vi "subVI_Mono2Go2Pos.vi"(2 "ESP300 Error":errorcluster, 3 "Postion (Unit)":dbl, 4 "ESP 300 COM Port":refnum<visa-resource-name>="COM4" caption="COM Port") -> (0 "error out":errorcluster, 1 "VISA resource name out":refnum<visa-resource-name>)   [LabVIEW 2019]
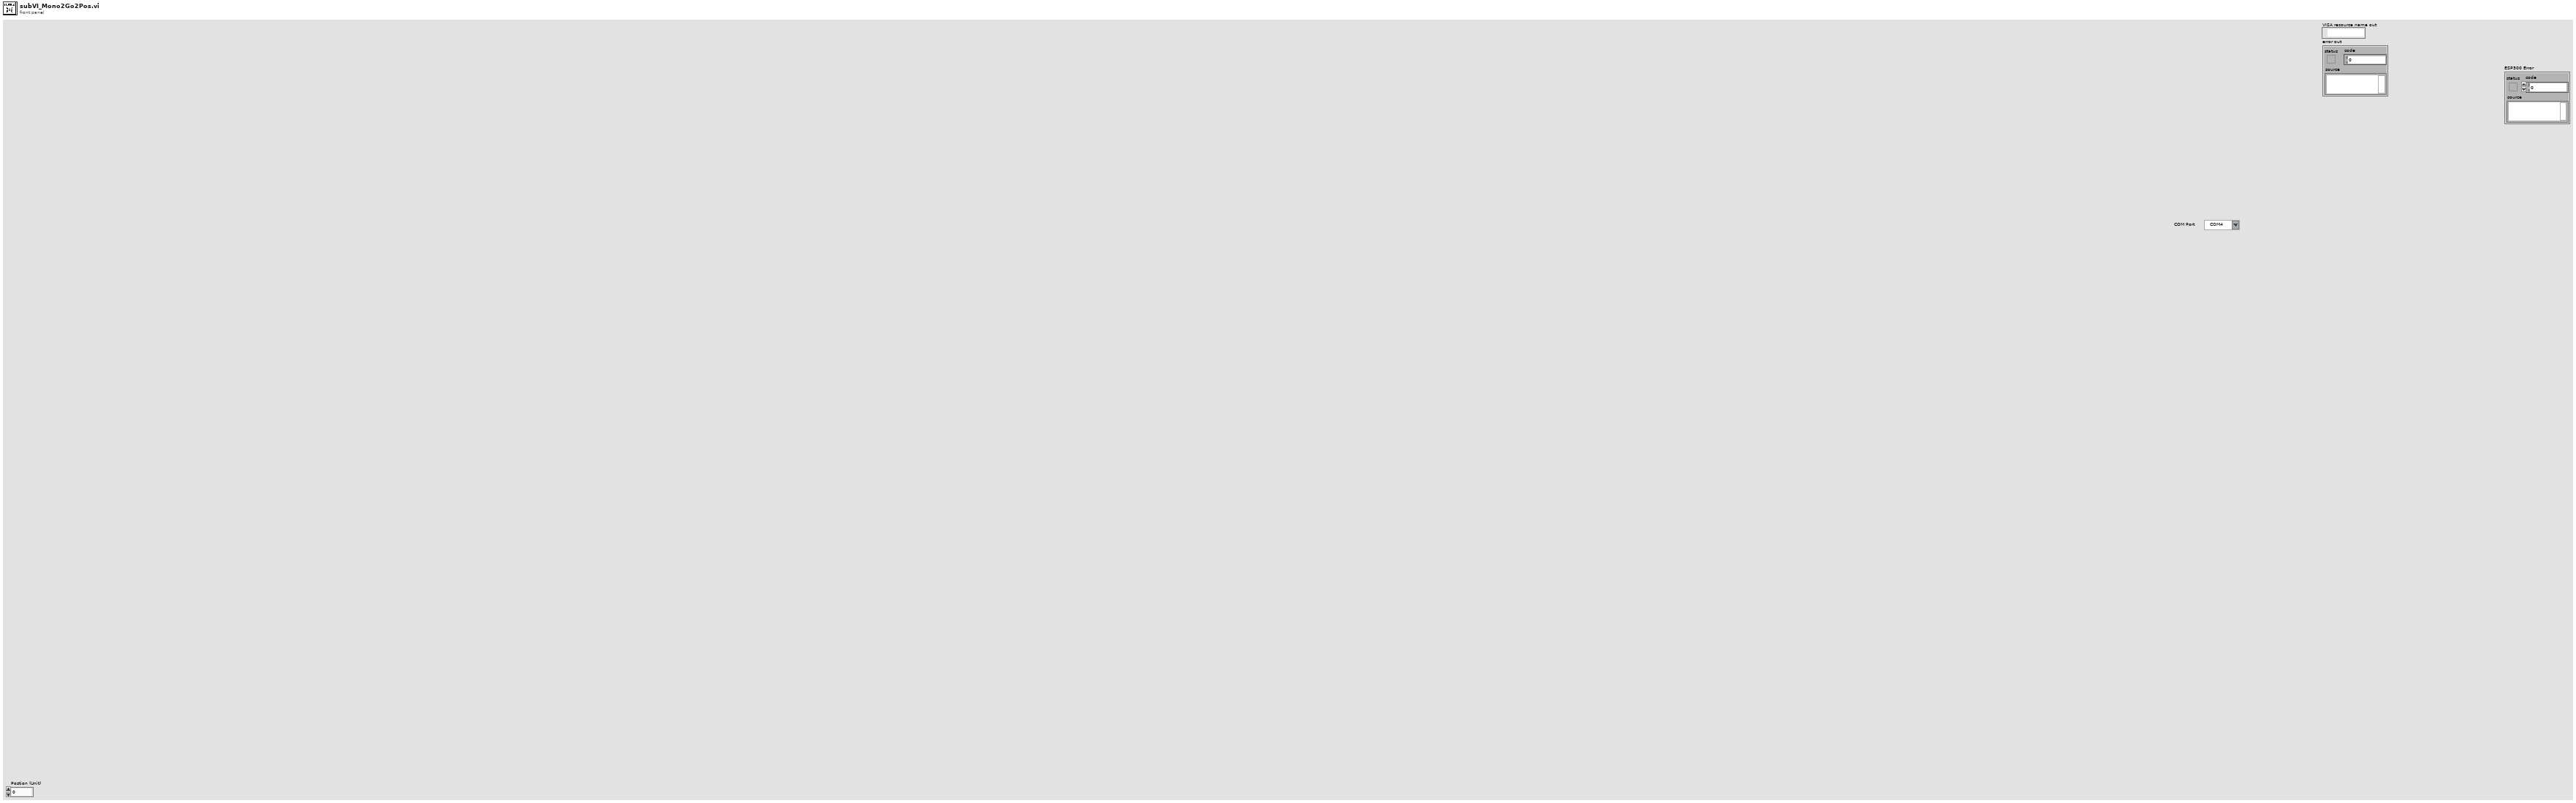
[diagram p1: front panel]
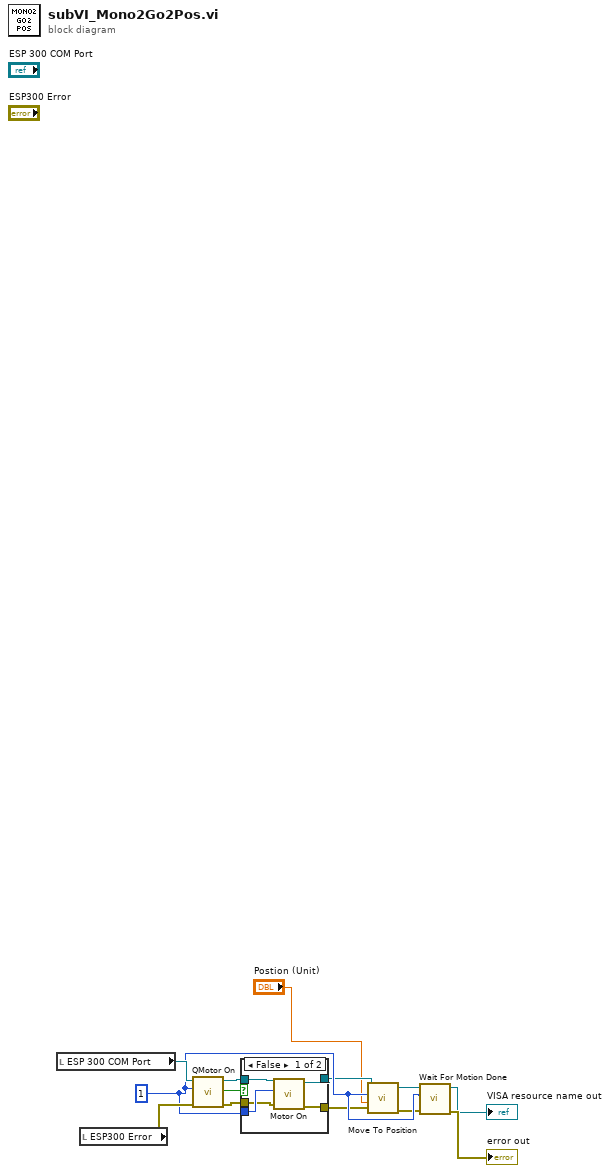
[diagram p0: block diagram]
diagram:
  w9 = 1 ("Axis")
  n1 = local read "ESP 300 COM Port"() -> (w11:refnum<visa-resource-name>)
  n2 = local read "ESP300 Error"() -> (w10:errorcluster)
  n3 = call "QMotor On.vi"("error in (no error)"=w10, "Axis"=w9, "VISA resource name in"=w11) -> ("error out"=w4:errorcluster, "Motor On?"=w2:bool, "VISA resource name out"=w3:refnum<visa-resource-name>)  [unwired: 6 in]
  n4 = case shown="False" w2 {
    tunnel: w9 -> [w18 _]
    tunnel: w3 -> [w17 w20]
    tunnel: w4 -> [w16 w19]
    tunnel: [w15 w20] -> w5
    tunnel: [w14 w19] -> w6
    frame False {
      n5 = call "Motor On.vi"("error in (no error)"=w16, "Axis"=w18, "VISA resource name in"=w17) -> ("error out"=w14:errorcluster, "VISA resource name out"=w15:refnum<visa-resource-name>)  [unwired: 7 in]
    }
    frame True {
    }
  }
  n6 = call "Move To Position.vi"("error in (no error)"=w6, "Postion (Unit)"="Postion (Unit)", "Axis"=w9, "VISA resource name in"=w5) -> ("error out"=w8:errorcluster, "VISA resource name out"=w7:refnum<visa-resource-name>)  [unwired: 6 in]
  n7 = call "Wait For Motion Done.vi"("error in (no error)"=w8, "Axis"=w9, "VISA resource name"=w7) -> ("error out"=→"error out":errorcluster, "VISA resource name out"=→"VISA resource name out":refnum<visa-resource-name>)  [unwired: 7 in]
